vi "BWC_analogSampleAveraged_sample_periodically.vi"(11 "Acquisition Time (s)":dbl=1.0 caption="Acquisition Time (s) (no change)") -> (0 "Error Out":errorcluster, 1 "size(s)":i32=20001)   [LabVIEW 2017]
uses:
  <vilib>/Analysis/2dsp.llb/Power Spectrum (DBL).vi
  <vilib>/VirtualBench/_MSO Configure Analog Channel0.vi
  <vilib>/VirtualBench/_MSO Configure Timing8.vi
  <vilib>/Utility/file.llb/Write Delimited Spreadsheet (DBL).vi
  <vilib>/VirtualBench/VirtualBench.lvlib
  <vilib>/Analysis/NI_AALBase.lvlib
  <vilib>/Analysis/NI_AALPro.lvlib
panel:
  out "path 2":path
  in  "postfix":string
  in  "prefix":string
  in  "path":string
  out "Analog Waveforms 2":waveform(dbl)(graph) caption="Analog Waveforms"
  in  "dark level":dbl
  out "(mean-darklvl)/std":dbl(graph)=0.019994885029411345
  out "std":dbl(graph)=0.019994885029411345
  out "mean-dark level":dbl(graph)=0.019994885029411345
  out "Analog Waveforms":waveform(dbl)[](graph)=[{"t0"=timestamp(3589833457.0102935 s since 1904-01-01), "dt"=5e-05, "Y"=array[20001 elements], "attributes"=variant("NI_ChannelName"=variant(string "mso/2"), "NI_UnitDescription"=variant(string "Volts"))}]
  in  "Auto Trigger":bool=TRUE caption="Auto Trigger (False)"
  in  "Pretrigger Time (s)":dbl=0.1 caption="Pretrigger Time (s) (no change)"
  in  "Sample Rate":dbl=20000.0 caption="Sample Rate (no change)"
  in  "Vertical Range":dbl=2.5 caption="Vertical Range (no change)"
  in  "Vertical Offset":dbl caption="Vertical Offset (no change)"
  in  "Probe Attenuation":i32(ring)=1 caption="Probe Attenuation (no change)" items=["1x"=1, "10x"=10]
  in  "Vertical Coupling":i32(ring)=1 caption="Vertical Coupling (no change)" items=["AC", "DC"]
  in  "Enable Channel":bool=TRUE caption="Enable Channel (no change)"
  in  "Channel":tag="mso/2"
  in  "Device Name":tag="VB8012-3059AE6"
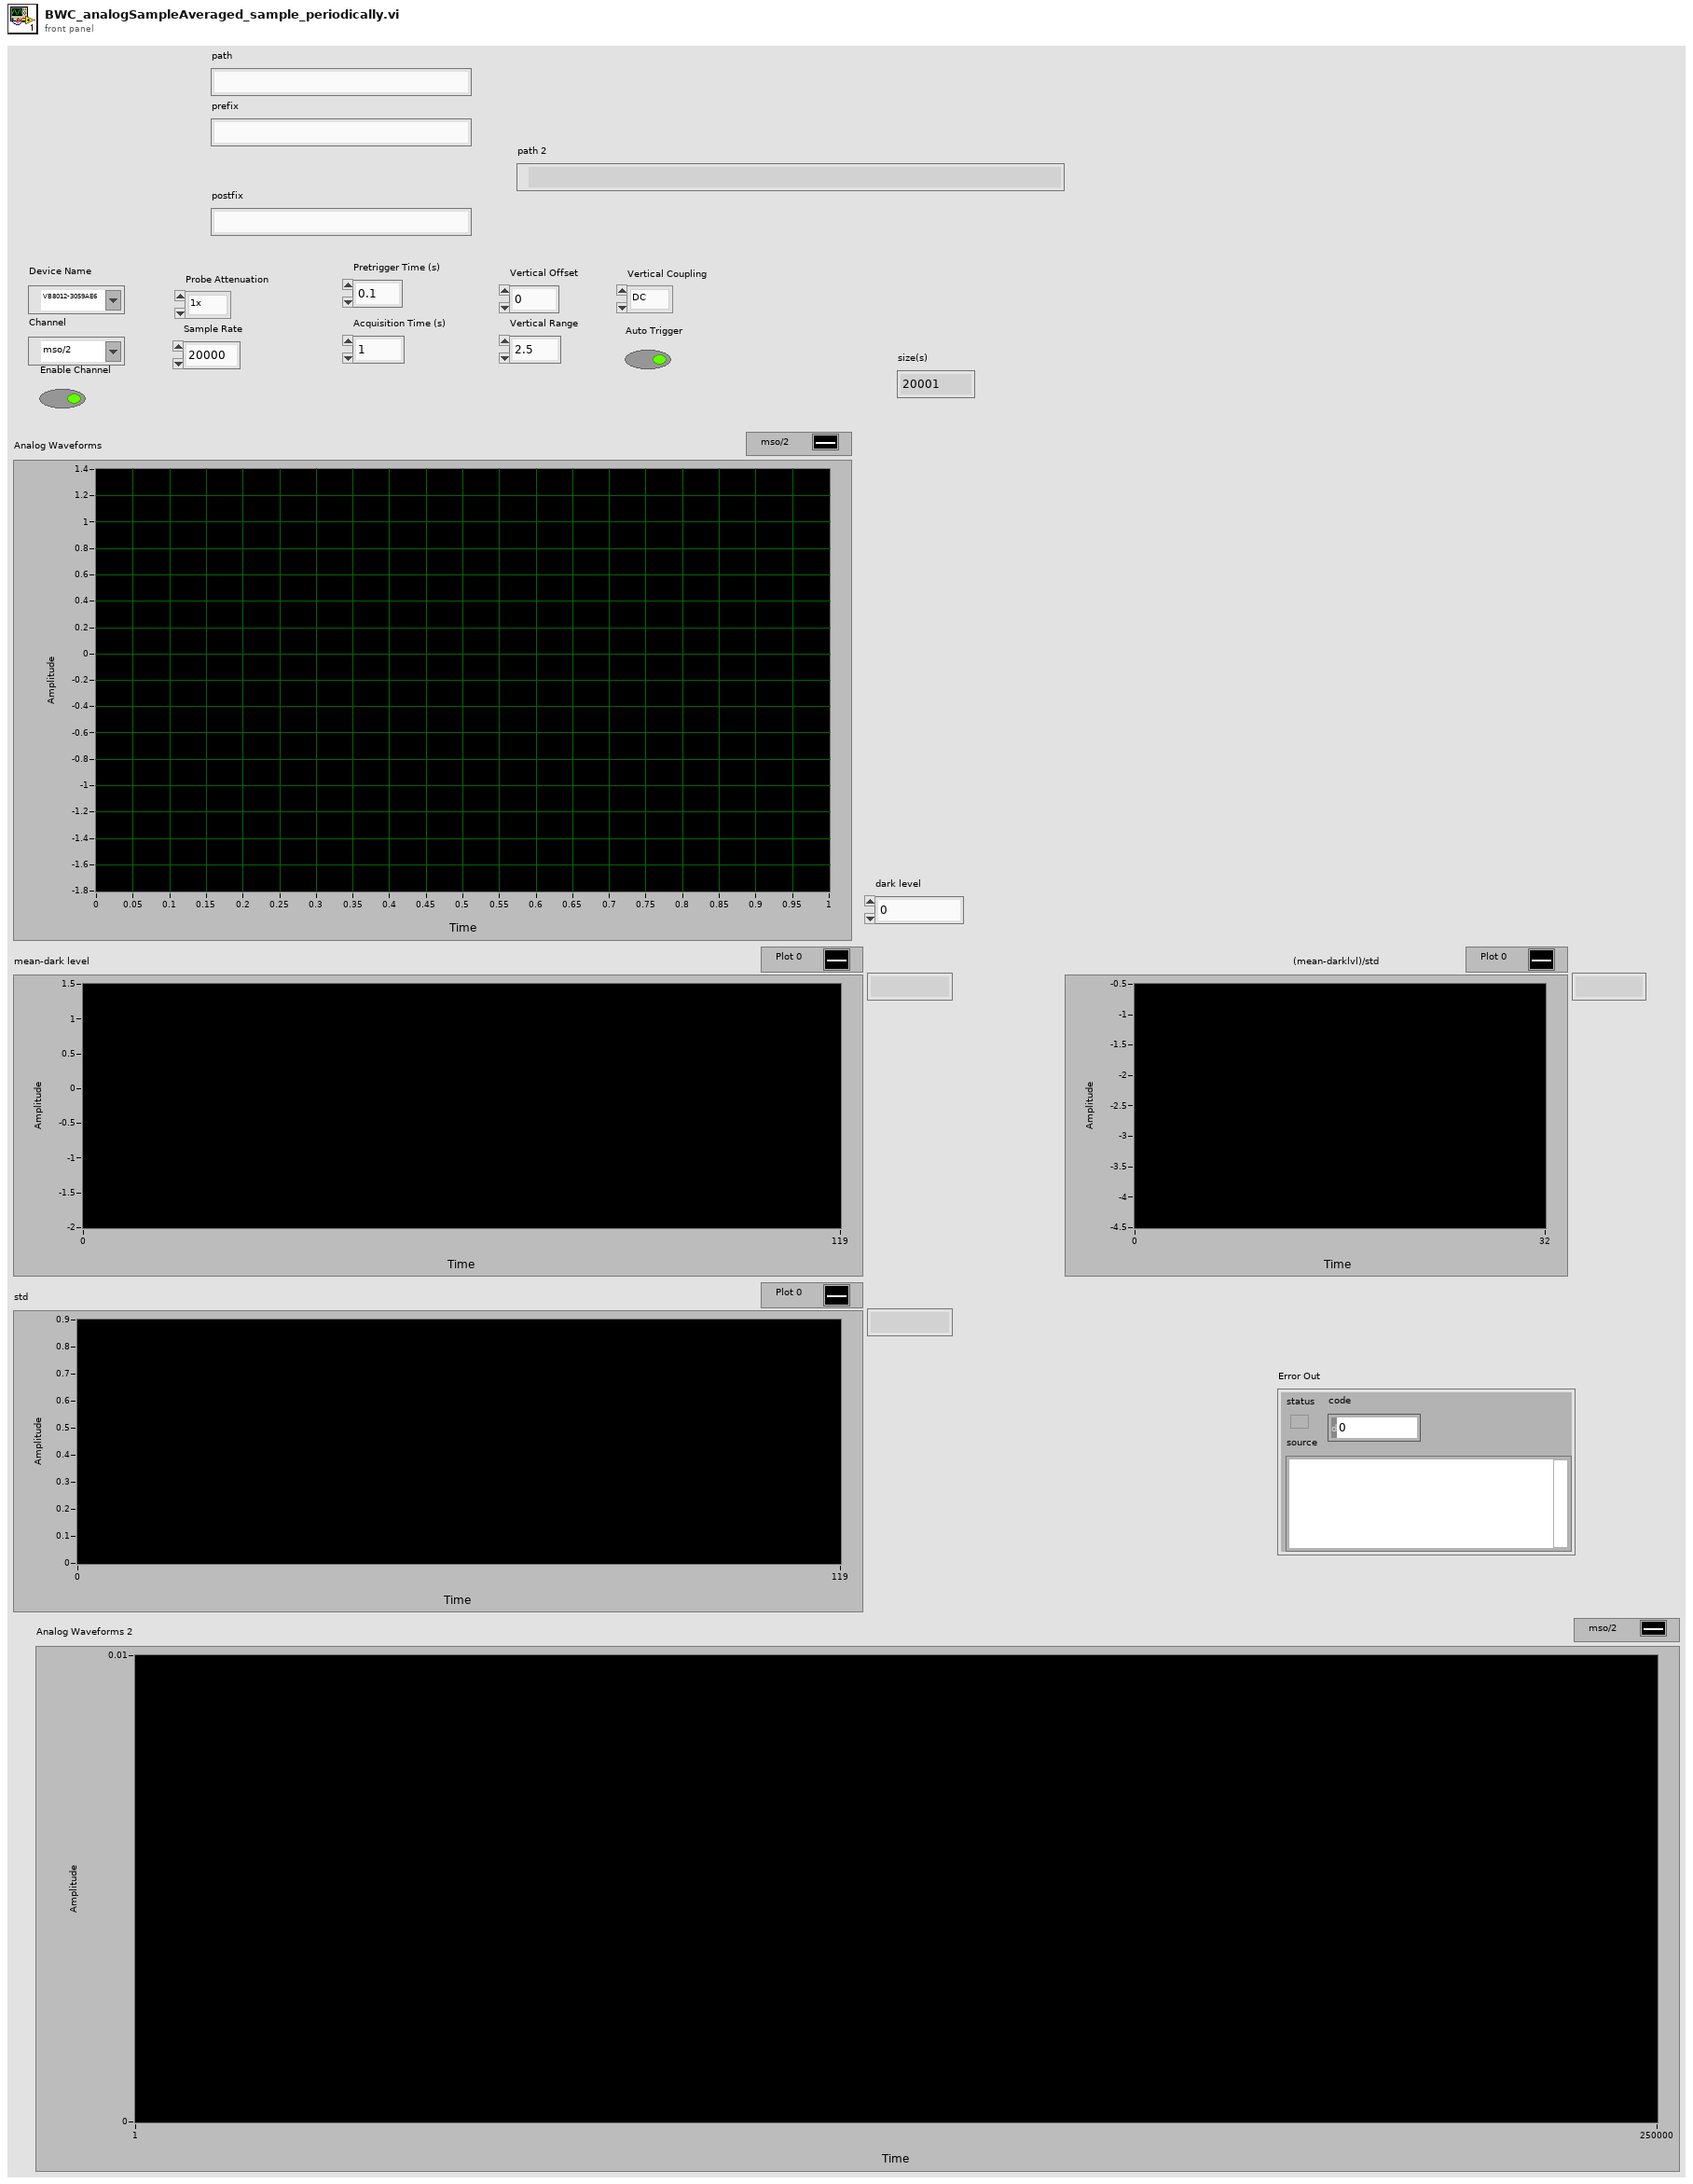
[diagram p1: front panel]
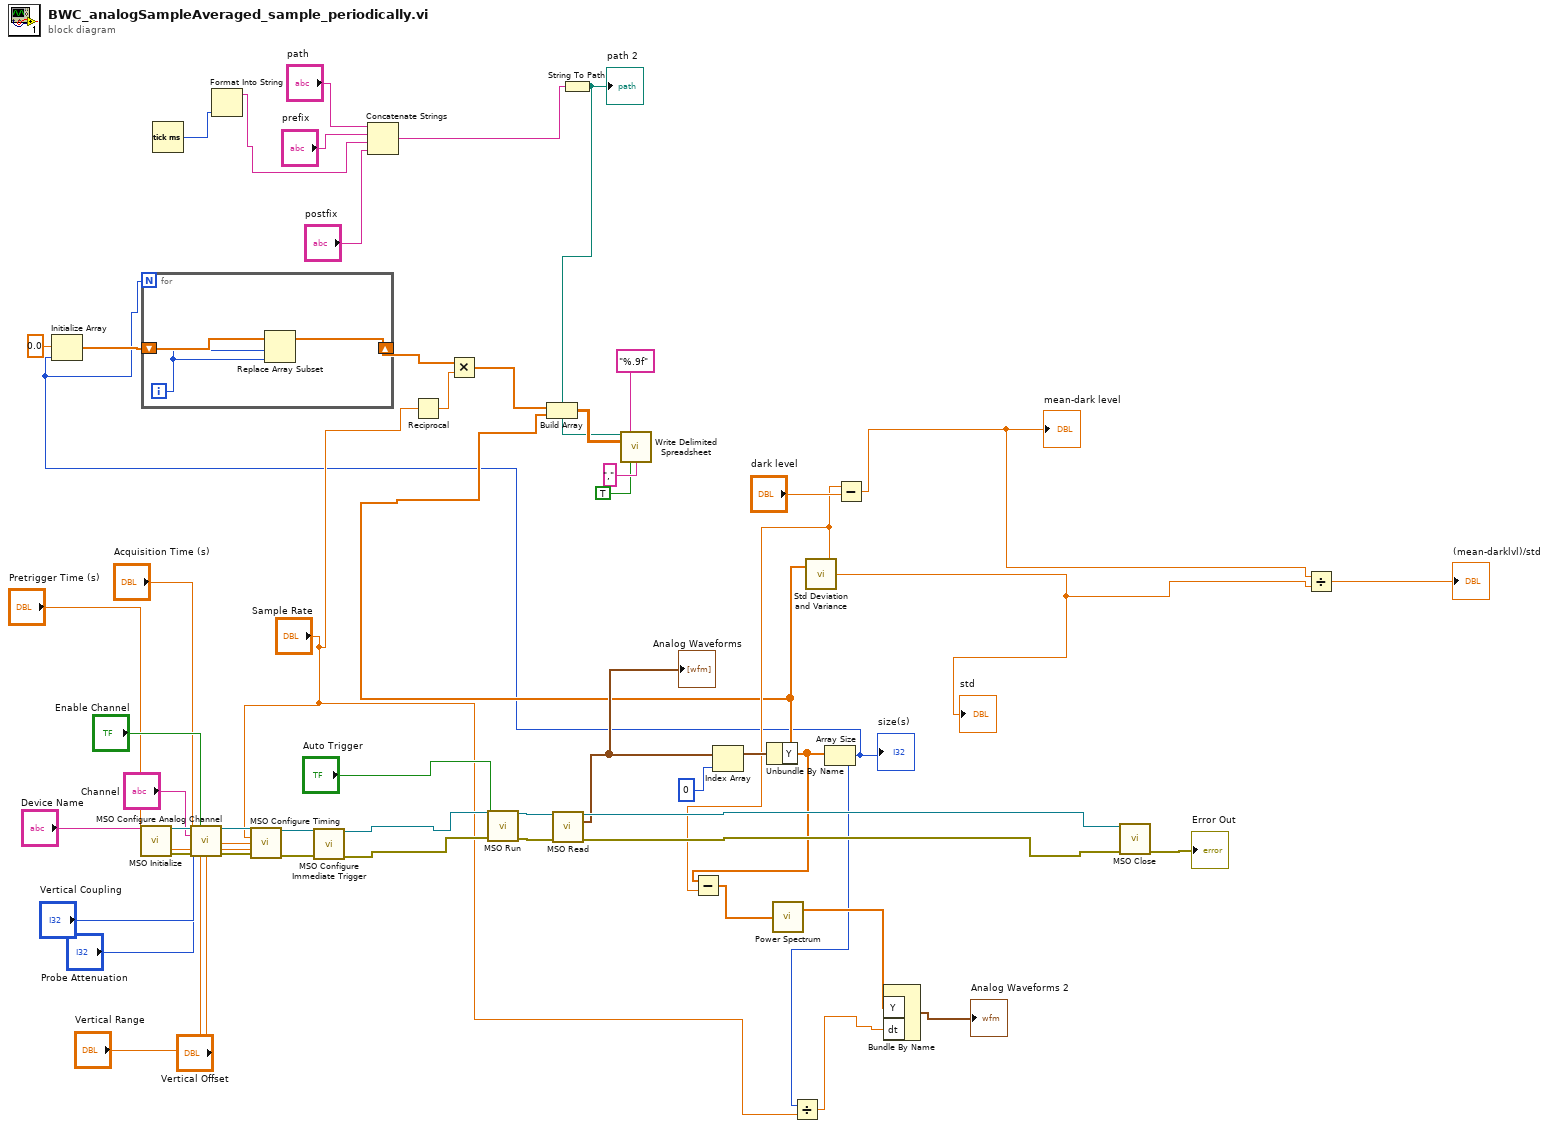
[diagram p0: block diagram]
diagram:
  n1 = call <vilib>:"MSO Initialize.vi"("Device Name"="Device Name") -> ("Instrument Handle Out"=w52:refnum<k21>, "Error Out"=w51:errorcluster)  [unwired: 13 in]
  n2 = Tick Count (ms)() -> (millisecond timer value=w3:u32)
  n3 = call-poly <vilib>:"MSO Configure Analog Channel.vi"("Instrument Handle In"=w52, "Enable Channel"="Enable Channel", "Channel"="Channel", "Vertical Coupling"="Vertical Coupling", "Probe Attenuation"="Probe Attenuation", "Error In"=w51, "Vertical Range"="Vertical Range", "Vertical Offset"="Vertical Offset") -> ("Instrument Handle Out"=w49:refnum<k21>, "Error Out"=w47:errorcluster)  [unwired: 6 in]
  n4 = Format Into String(w3) -> (resulting string=w2:string)  [unwired: 3 in, 1 out]
  n5 = call-poly <vilib>:"MSO Configure Timing.vi"("Instrument Handle In"=w49, "Sample Rate"="Sample Rate", "Acquisition Time (s)"="Acquisition Time (s)", "Pretrigger Time (s)"="Pretrigger Time (s)", "Error In"=w47) -> ("Instrument Handle Out"=w48:refnum<k21>, "Error Out"=w46:errorcluster)  [unwired: 9 in]
  n6 = call <vilib>:"MSO Configure Immediate Trigger.vi"("Instrument Handle In"=w48, "Error In"=w46) -> ("Instrument Handle Out"=w33:refnum<k21>, "Error Out"=w34:errorcluster)  [unwired: 12 in]
  n7 = Concatenate Strings("path", "prefix", w2, "postfix") -> (w4:string)
  n8 = Reciprocal(x="Sample Rate") -> (1/x=w15:dbl)
  n9 = call <vilib>:"MSO Run.vi"("Instrument Handle In"=w33, "Auto Trigger"="Auto Trigger", "Error In"=w34) -> ("Instrument Handle Out"=w38:refnum<k21>, "Error Out"=w37:errorcluster)  [unwired: 11 in]
  n10 = call <vilib>:"MSO Read.vi"("Instrument Handle In"=w38, "Error In"=w37) -> ("Instrument Handle Out"=w30:refnum<k21>, "Analog Waveforms"=w20:waveform(dbl)[], "Error Out"=w31:errorcluster)  [unwired: 8 in, 3 out]
  "Analog Waveforms" <- w20
  n11 = String To Path(string=w4) -> (path=w1:path)
  "path 2" <- w1
  n12 = Index Array(array=w20, index=0) -> (element=w35:waveform(dbl))
  n13 = Unbundle By Name(w35) -> ("Y"=w13:dbl[])
  n14 = call <vilib>:"Std Deviation and Variance.vi"("X"=w13) -> ("mean"=w24:dbl, "standard deviation"=w22:dbl)  [unwired: 1 in, 1 out]
  "std" <- w22
  n15 = Subtract(x=w13, y=w24) -> (x-y=w23:dbl[])
  n16 = call-poly <vilib>:"Power Spectrum.vi"("X"=w23) -> ("Power Spectrum"=w27:dbl[])  [unwired: 1 out]
  n17 = Array Size(array=w13) -> (size(s)=w12:i32)
  "size(s)" <- w12
  n18 = Initialize Array(0.0 ("element"), w12) -> (w18:dbl[])
  n19 = for {
    N: w12 -> [_]
    shift-right: [w55] -> w17
    shift-left: w18 -> [w57]
    i -> [w56]
    n20 = Replace Array Subset(array=w57, new element=w56, index=w56) -> (w55:dbl[])
  }
  n21 = Multiply(x=w17, y=w15) -> (x*y=w14:dbl[])
  n22 = Build Array(w14, w13) -> (w11:dbl[][])
  n23 = call-poly <vilib>:"Write Delimited Spreadsheet.vi"("file path (dialog if empty)"=w1, "format (%.3f)"="%.9f", "2D data"=w11, "transpose? (no:F)"=TRUE, "delimiter (\\t)"="," ("delimiter (\\t)")) -> ()  [unwired: 9 in, 2 out]
  n24 = Divide(x=w12, y="Sample Rate") -> (x/y=w25:dbl)
  n25 = Subtract(x=w24, y="dark level") -> (x-y=w21:dbl)
  "mean-dark level" <- w21
  n26 = Bundle By Name("Y"=w27, "dt"=w25) -> (→"Analog Waveforms 2":waveform(dbl))  [unwired: 1 in]
  n27 = call <vilib>:"MSO Close.vi"("Instrument Handle In"=w30, "Error In"=w31) -> ("Error Out"=→"Error Out":errorcluster)  [unwired: 13 in]
  n28 = Divide(x=w21, y=w22) -> (x/y=→"(mean-darklvl)/std":dbl)
